vi "Disconnect PV.vi"(8 "error in (no error)":errorcluster, 10 "PV URL":string, 11 "CS++DSMonitor in":refnum<class "CS++DSMonitor.lvclass">) -> (0 "error out":errorcluster, 3 "CS++DSMonitor out":refnum<class "CS++DSMonitor.lvclass">)   [LabVIEW 2015, in "CS++DSMonitor.lvlib" / "CS++DSMonitor.lvclass"]
doc: "Close connection to process variable."
uses:
  CS++DSMonitor.lvclass
  CS++PVMonitor/CS++PVMonitor.lvclass/CS++PVMonitor.ctl
  CS++DSMonitor.lvclass/CS++DSMonitor.ctl
  CS++PVMonitor/CS++PVMonitor.lvclass
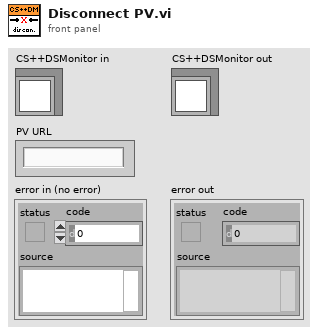
[diagram p1: front panel]
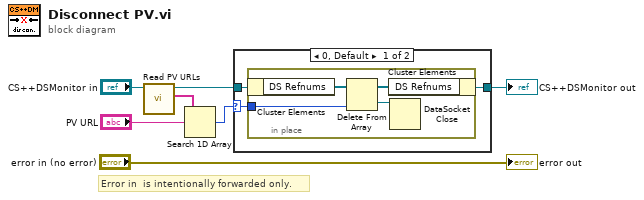
[diagram p0: block diagram]
diagram:
  # "Error in  is intentionally forwarded only."
  n1 = call "Read PV URLs.vi"("CS++PVMonitor in"="CS++DSMonitor in") -> ("PV URLs"=w6:string[], "CS++PVMonitor out"=w3:refnum<class "CS++DSMonitor.lvclass">)  [unwired: 8 in, 1 out]
  n2 = Search 1D Array(1D array=w6, element="PV URL") -> (index of element=w4:i32)  [unwired: 1 in]
  n3 = case shown="0, Default" w4 {
    selector: w4 -> [w10 _]
    tunnel: w3 -> [w9 w15]
    tunnel: [w8 w15] -> w2
    frame 0, Default {
      n4 = in-place {
        in-place-border: w10 -> [w12]
        n5 = in-place-cluster #1(w9) -> ("DS Refnums"=w14:refnum<k13>[])
        n6 = Delete From Array(array=w14, index=w12) -> (deleted portion=w11:refnum<k13>, array with subset deleted=w13:refnum<k13>[])  [unwired: 1 in]
        n7 = in-place-cluster #1("DS Refnums"=w13) -> (w8:refnum<class "CS++DSMonitor.lvclass">)
        n8 = DataSocket Close(11:w11) -> ()  [unwired: 2 in, 2 out]
      }
    }
    frame -1 {
    }
  }
  "CS++DSMonitor out" <- w2
  "error out" <- "error in (no error)"
